vi "UI - Preferences.vi"() -> ()   [LabVIEW 2020, in "cycling structure demo UI.lvlib" / "Configuration.lvclass"]
doc: "Module UI that appears in the Configuration UI.\n____\nPeloton Config 2.0.0.6\nCopyright (c) 2024, Peloton"
uses:
  Configuration.lvclass
  <vilib>/Peloton/Peloton Config/DCFG Framework/Init UI Params--cluster.ctl
  <vilib>/Peloton/Peloton Config/DCFG Framework/Configuration_class/Configuration.lvclass
  <vilib>/Peloton/Peloton Config/DCFG Framework/Stop Argument--cluster.ctl
  <vilib>/Peloton/Peloton Config/DCFG Framework/Send Config to Page Argument--cluster.ctl
  <vilib>/Peloton/Peloton Config/DCFG Framework/Send Stop to Page Argument--cluster.ctl
  C:/Program Files (x86)/National Instruments/LabVIEW 2020/vi.lib/Peloton/Peloton Config/DCFG Framework/Configuration_class/Configuration.lvclass
  <vilib>/Peloton/Peloton Config/DCFG Framework/Configuration_class/Configuration.lvclass/Configuration.ctl
  Configuration--cluster.ctl
  Configuration.lvclass/Configuration.ctl
  Set Configuration.vi
  Get Configuration.vi
  <vilib>/Peloton/Peloton Config/DCFG Framework/Configuration_class/Get Name.vi
  <vilib>/Peloton/Peloton Config/DCFG Framework/Peloton_lib_DCFG Framework.lvlib
panel:
  in  "Random Path":path
  in  "Init UI Params":T1
  # "Define the Default Configuration UI here."
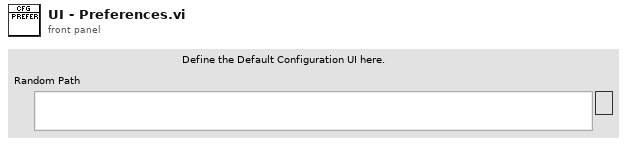
[diagram p1: front panel]
types:
  T1 = typedef "Peloton_lib_DCFG Framework.lvlib/Init UI Params--cluster.ctl" = cluster{"Initial Config":refnum<class "Configuration.lvclass">, "Stop CFG Module":refnum<user-event>, "Send Config to Page":refnum<user-event>, "Send Stop to Page":refnum<user-event>, "Reset Page Defaults":refnum<user-event>}
  T2 = enum32{"Invalid", "Standard", "Closed", "Hidden", "Minimized", "Maximized"}
  T3 = typedef "cycling structure demo UI.lvlib/Configuration.lvclass/Configuration--cluster.ctl" = cluster{"Random Path":path}
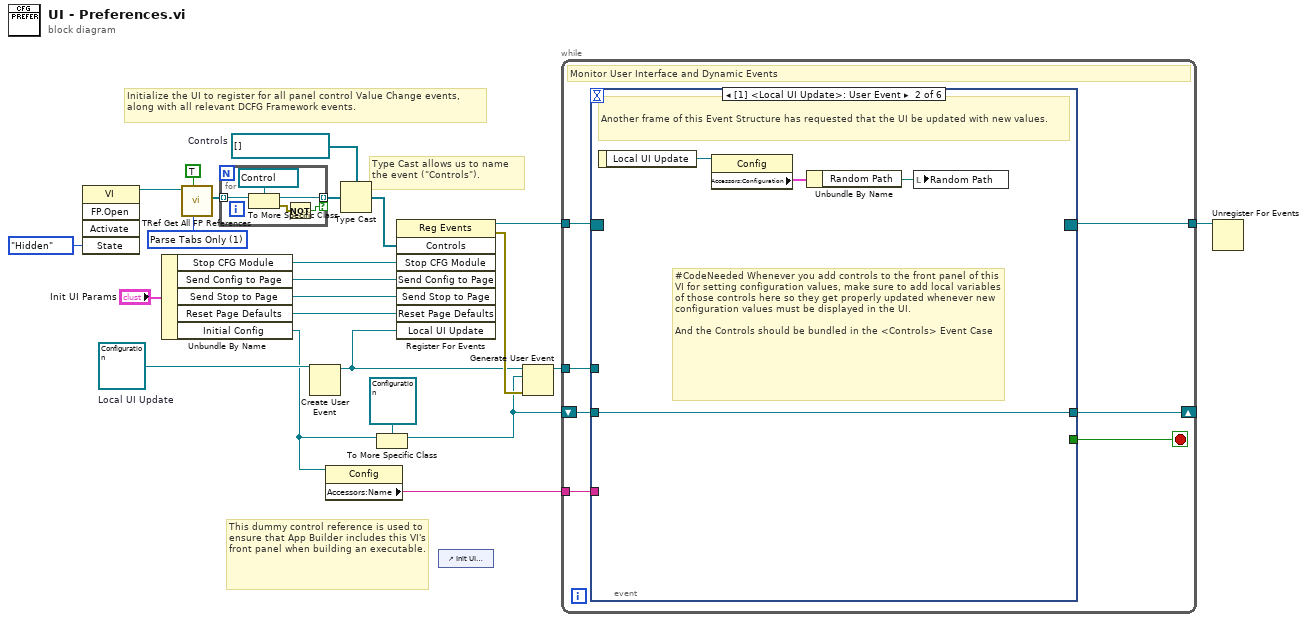
[diagram p0: block diagram]
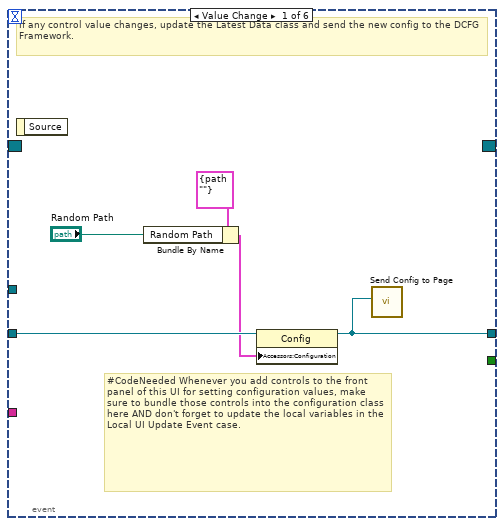
[diagram p2: hidden frame]
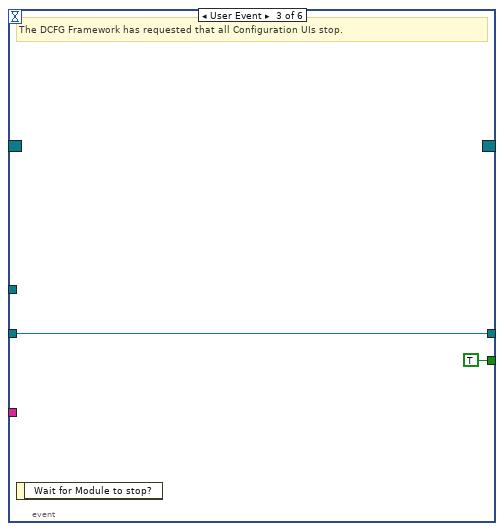
[diagram p3: hidden frame]
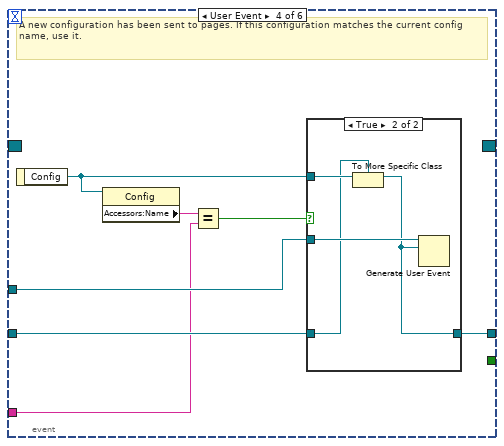
[diagram p4: hidden frame]
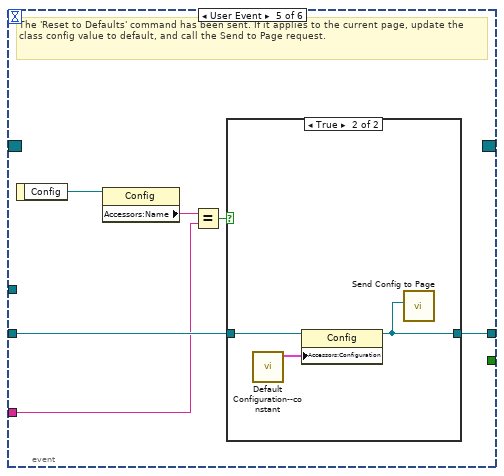
[diagram p6: hidden frame]
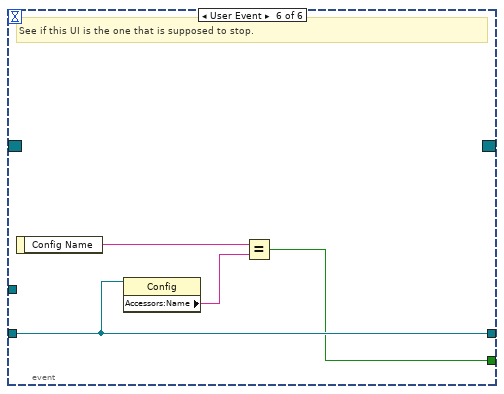
[diagram p8: hidden frame]
diagram:
  w3 = refnum<vi>[] []  # Controls
  w9 = u16 1 items=["Parse All", "Parse Tabs Only"] ("Parsing Rule")
  w20 = refnum<class "Configuration.lvclass"> refnum  # Local UI Update
  # "Type Cast allows us to name the event (\"Controls\")."
  # "Initialize the UI to register for all panel control Value Change events, along with all relevant DCFG Framework events."
  # "This dummy control reference is used to ensure that App Builder includes this VI's front panel when building an executable."
  n1 = invoke on="Invoke Node" class="VI" method="FP.Open"("State"=T2."Hidden") -> (reference out=w8:refnum<vi>)  [unwired: 4 in, 4 out]
  n2 = Unbundle By Name("Init UI Params") -> ("Stop CFG Module"=w16:refnum<user-event>, "Send Config to Page"=w15:refnum<user-event>, "Send Stop to Page"=w14:refnum<user-event>, "Reset Page Defaults"=w13:refnum<user-event>, "Initial Config"=w5:refnum<class "Configuration.lvclass">)
  n3 = call <vilib>:"TRef Get All FP References.vi"("Parsing Rule"=w9, "Ignore Decorations?"=TRUE, "VI Refnum"=w8) -> ("All FP Objects"=w10:refnum<vi>[])  [unwired: 4 in, 4 out]
  n4 = for {
    tunnel: w10 -> [w28] mode=indexing
    tunnel: [w27] -> w2 mode=indexing if=w24
    n5 = To More Specific Class(target class=refnum<vi> refnum ("Controls"), reference=w28) -> (specific class reference=w27:refnum<vi>, error out=w25:errorcluster)  [unwired: 1 in]
    n6 = Not(x=w25) -> (.not. x?=w24:bool)
  }
  n7 = Create User Event(user event datatype=w20) -> (user event=w12:refnum<user-event>)  [unwired: 1 in, 1 out]
  n8 = property class="Config"(reference=w5) -> ("Accessors:Name"=w4:string)  [unwired: 1 in, 2 out]
  n9 = Type Cast(type=w3, x=w2) -> (*(type *) &x=w1:refnum<vi>[])
  n10 = To More Specific Class(target class=refnum<class "Configuration.lvclass"> refnum ("Sample Module 1.lvlib:Config"), reference=w5) -> (specific class reference=w7:refnum<class "Configuration.lvclass">)  [unwired: 1 in, 1 out]
  n11 = register-events(w1, w16, w15, w14, w13, w12) -> (reference out=w22:refnum<event-registration>, error out=w18:errorcluster)  [unwired: 2 in]
  n12 = control-ref of="Init UI Params"() -> ()  [unwired: 1 out]
  n13 = Generate User Event(user event=w12, event data cluster=w7, error in=w18) -> (user event out=w19:refnum<user-event>)  [unwired: 1 in, 1 out]
  n14 = while {
    tunnel: w22 -> [w35]
    tunnel: [w34] -> w21
    shift-right: [w30] -> _
    shift-left: w7 -> [w33]
    tunnel: w19 -> [w31]
    tunnel: w4 -> [w29]
    stop <- w32 stop-if-true
    # "Monitor User Interface and Dynamic Events"
    n15 = event shown="[1] <Local UI Update>: User Event" {
      selector: w35 -> [_ _ _ _ _ _]
      dyn-events: [_ _ _ _ _ _] -> w34
      timeout: _ -> [_ _ _ _ _ _]
      tunnel: w33 -> [w39 w44 w46 w51 w63 w72]
      tunnel: [w38 w44 w46 w52 w64 w72] -> w30
      tunnel: [_ _ TRUE ("Addressed to this instance?") _ _ w69] -> w32
      tunnel: w31 -> [_ _ _ w53 _ _]
      tunnel: w29 -> [_ _ _ w48 w60 _]
      event Value Change {
        # "#CodeNeeded Whenever you add controls to the front panel of this UI for setting configuration values, make sure to bundle those controls into the configuration class here AND don't forget to update the local variables in the Local UI Update Event case."
        # "If any control value changes, update the Latest Data class and send the new config to the DCFG Framework."
        n16 = event-data() -> ()  [unwired: 1 in, 1 out]
        n17 = Bundle By Name(cluster=T3 {"Random Path"=path ""} ("Configuration"), "Random Path"="Random Path") -> (w37:T3)
        n18 = property class="Config"(reference=w39, "Accessors:Configuration"=w37) -> (reference out=w38:refnum<class "Configuration.lvclass">)  [unwired: 1 in, 1 out]
        n19 = call <vilib>:"Send Config to Page.vi"("Config"=w38) -> ()  [unwired: 10 in, 1 out]
      }
      event User Event {
        # "#CodeNeeded Whenever you add controls to the front panel of this VI for setting configuration values, make sure to add local variables of those controls here so they get properly updated whenever new configuration values must be displayed in the UI.\n\nAnd the Controls should be bundled in the <Controls> Event Case"
        # "Another frame of this Event Structure has requested that the UI be updated with new values."
        n20 = event-data() -> ("Local UI Update"=w43:refnum<class "Configuration.lvclass">)  [unwired: 1 in]
        n21 = property class="Config"(reference=w43) -> ("Accessors:Configuration"=w42:T3)  [unwired: 1 in, 2 out]
        n22 = Unbundle By Name(w42) -> ("Random Path"=w41:path)
        n23 = local write "Random Path"(w41) -> ()
      }
      event User Event {
        # "The DCFG Framework has requested that all Configuration UIs stop."
        n24 = event-data() -> ()  [unwired: 1 in, 1 out]
      }
      event User Event {
        # "A new configuration has been sent to pages. If this configuration matches the current config name, use it."
        n25 = event-data() -> ("Config"=w50:refnum<class "Configuration.lvclass">)  [unwired: 1 in]
        n26 = property class="Config"(reference=w50) -> ("Accessors:Name"=w49:string)  [unwired: 1 in, 2 out]
        n27 = Equal?(x=w49, y=w48) -> (x = y?=w47:bool)
        n28 = case shown="True" w47 {
          tunnel: w53 -> [_ w58]
          tunnel: w51 -> [w54 w55]
          tunnel: [w54 w57] -> w52
          tunnel: w50 -> [_ w56]
          frame False {
          }
          frame True {
            n29 = To More Specific Class(target class=w55, reference=w56) -> (specific class reference=w57:refnum<class "Configuration.lvclass">)  [unwired: 1 in, 1 out]
            n30 = Generate User Event(user event=w58, event data cluster=w57) -> ()  [unwired: 2 in, 2 out]
          }
        }
      }
      event User Event {
        # "The 'Reset to Defaults' command has been sent. If it applies to the current page, update the class config value to default, and call the Send to Page request."
        n31 = event-data() -> ("Config"=w62:refnum<class "Configuration.lvclass">)  [unwired: 1 in]
        n32 = property class="Config"(reference=w62) -> ("Accessors:Name"=w61:string)  [unwired: 1 in, 2 out]
        n33 = Equal?(x=w61, y=w60) -> (x = y?=w59:bool)
        n34 = case shown="True" w59 {
          tunnel: w63 -> [w65 w68]
          tunnel: [w65 w66] -> w64
          frame False {
          }
          frame True {
            n35 = call "Default Configuration--constant.vi"() -> ("Default Configuration"=w67:T3)  [unwired: 11 in]
            n36 = property class="Config"(reference=w68, "Accessors:Configuration"=w67) -> (reference out=w66:refnum<class "Configuration.lvclass">)  [unwired: 1 in, 1 out]
            n37 = call <vilib>:"Send Config to Page.vi"("Config"=w66) -> ()  [unwired: 10 in, 1 out]
          }
        }
      }
      event User Event {
        # "See if this UI is the one that is supposed to stop."
        n38 = event-data() -> ("Config Name"=w71:string)  [unwired: 1 in]
        n39 = property class="Config"(reference=w72) -> ("Accessors:Name"=w70:string)  [unwired: 1 in, 2 out]
        n40 = Equal?(x=w71, y=w70) -> (x = y?=w69:bool)
      }
    }
  }
  n41 = Unregister For Events(event registration refnum=w21) -> ()  [unwired: 1 in, 1 out]
